vi "DIAG_STM Write Meta Data.vi"   [LabVIEW 2013, in "Diagnostics Addon Engine.lvlib"]
doc: "Use this VI to transmit the meta data cluster to a remote computer. Sending the meta data to another computer helps maintainability since the data resides only on one side and it is shared to other computers at run time."
uses:
  Diagnostics Addon Engine.lvlib
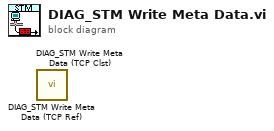
[diagram p0: block diagram]
diagram:
  n1 = call "DIAG_STM Write Meta Data (TCP Ref).vi"() -> ()  [unwired: 10 in, 2 out]
  n2 = call "DIAG_STM Write Meta Data (TCP Clst).vi"() -> ()  [unwired: 10 in, 2 out]
